vi "Generate Keithley DMM7510 Data.vi"(7 "Previous End":i32, 8 "error in (no error)":errorcluster, 11 "VISA resource name in":refnum<visa-resource-name>) -> (0 "error out":errorcluster, 2 "Graph Data":waveform(dbl)[](array[waveform]), 3 "VISA resource name out":refnum<visa-resource-name>, 4 "Actual sampling time (mean)":dbl, 5 "Current End":i32)   [LabVIEW 2017, in "Acquisition.lvlib"]
doc: "Generates sample waveforms according to the signal type in the HW Config input."
uses:
  Acquisition.lvlib
  <vilib>/Analysis/baseanly.llb/Mean (DBL).vi
  <vilib>/Analysis/NI_AALBase.lvlib
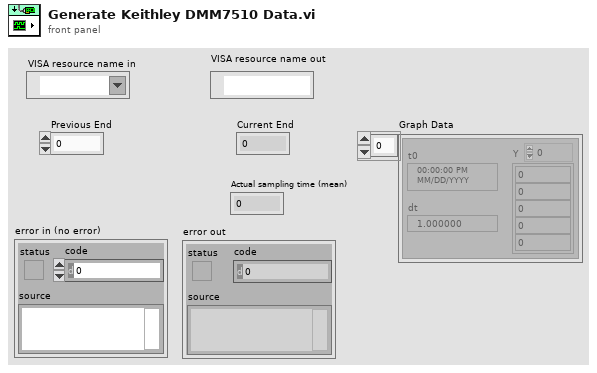
[diagram p1: front panel]
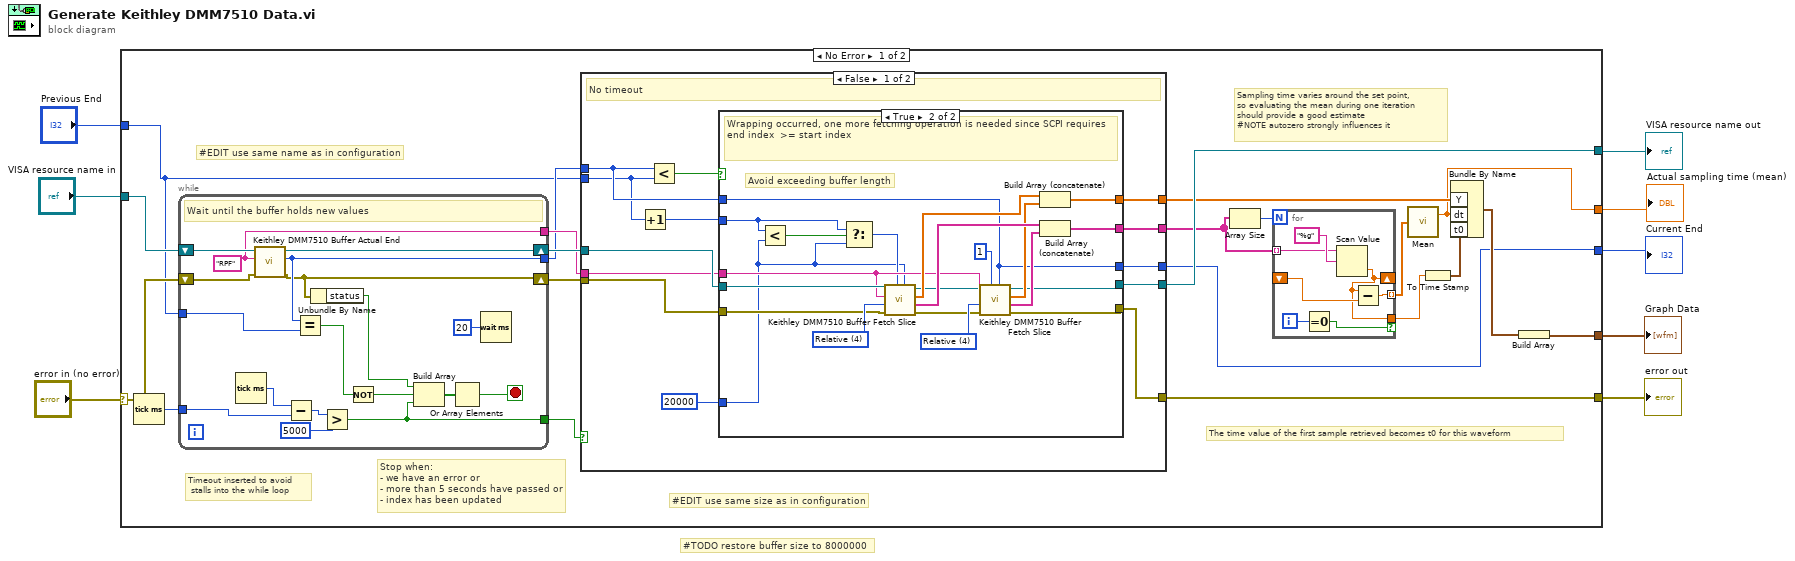
[diagram p0: block diagram]
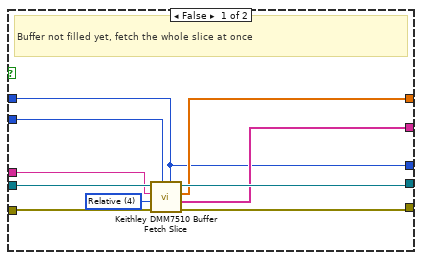
[diagram p2: hidden frame]
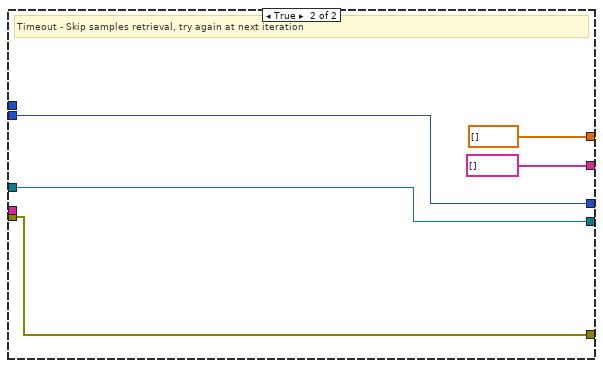
[diagram p3: hidden frame]
diagram:
  # "#TODO restore buffer size to 8000000"
  n1 = case shown="No Error" "error in (no error)" {
    selector: "error in (no error)" -> [w24 w105]
    tunnel: [w22 w105] -> w7
    tunnel: "VISA resource name in" -> [w25 w104]
    tunnel: [w21 w104] -> w5
    tunnel: "Previous End" -> [w23 _]
    tunnel: [w18 _] -> w3
    tunnel: [w17 _] -> w2
    tunnel: [w10 _] -> w1
    frame No Error {
      # "The time value of the first sample retrieved becomes t0 for this waveform"
      # "#EDIT use same name as in configuration"
      # "#EDIT use same size as in configuration"
      # "Timeout inserted to avoid\n stalls into the while loop"
      # "Stop when:\n- we have an error or\n- more than 5 seconds have passed or\n- index has been updated"
      # "Sampling time varies around the set point,\nso evaluating the mean during one iteration\nshould provide a good estimate\n#NOTE autozero strongly influences it"
      n2 = Tick Count (ms)() -> (millisecond timer value=w9:u32)
      n3 = while {
        shift-right: [w46] -> w29
        shift-left: w25 -> [w47]
        shift-right: [w41] -> w28
        shift-left: w24 -> [w45]
        tunnel: [w44] -> w27
        tunnel: [w43] -> w26
        tunnel: w23 -> [w42]
        tunnel: w9 -> [w38]
        tunnel: [w31] -> w14
        stop <- w40 stop-if-true
        w44 = "RPF" ("Buffer Name (defbuffer1)")
        # "Wait until the buffer holds new values"
        n4 = Tick Count (ms)() -> (millisecond timer value=w39:u32)
        n5 = call "Keithley DMM7510 Buffer Actual End.vi"("error in (no error)"=w45, "Buffer Name (defbuffer1)"=w44, "VISA resource name"=w47) -> ("error out"=w41:errorcluster, "Actual End"=w43:i32, "VISA resource name out"=w46:refnum<visa-resource-name>)  [unwired: 6 in]
        n6 = Subtract(x=w39, y=w38) -> (x-y=w37:u32)
        n7 = Equal?(x=w43, y=w42) -> (x = y?=w34:bool)
        n8 = Unbundle By Name(w41) -> ("status"=w32:bool)
        n9 = Greater?(x=w37, y=u32 5000) -> (0:w31:bool)
        n10 = Not(x=w34) -> (.not. x?=w33:bool)
        n11 = Build Array(w32, w33, w31) -> (w35:bool[])
        n12 = Or Array Elements(Boolean array=w35) -> (logical OR=w40:bool)
        n13 = Wait (ms)(milliseconds to wait=u32 20) -> ()  [unwired: 1 out]
      }
      n14 = case shown="False" w14 {
        tunnel: w29 -> [w59 w95]
        tunnel: w28 -> [w58 w96]
        tunnel: w27 -> [w57 _]
        tunnel: w26 -> [w56 _]
        tunnel: w23 -> [w53 w94]
        tunnel: [w52 w96] -> w22
        tunnel: [w51 w95] -> w21
        tunnel: [w50 dbl[] [] ("Measurements")] -> w20
        tunnel: [w49 w94] -> w17
        tunnel: [w48 string[] [] ("Element Value")] -> w15
        frame False {
          # "No timeout"
          n15 = Increment(x=w53) -> (x+1=w55:i32)
          n16 = Less?(x=w56, y=w53) -> (x < y?=w60:bool)
          n17 = case shown="True" w60 {
            tunnel: w58 -> [w69 w80]
            tunnel: w57 -> [w68 w83]
            tunnel: w59 -> [w70 w91]
            tunnel: 20000 ("Buffer Size") -> [_ w72]
            tunnel: [w66 w76] -> w51
            tunnel: [w65 w78] -> w52
            tunnel: [w62 w75] -> w49
            tunnel: w55 -> [w67 w71]
            tunnel: [w64 w90] -> w50
            tunnel: [w63 w89] -> w48
            tunnel: w56 -> [w62 w75]
            frame False {
              w61 = u16 4 items=["Date", "Extra", "Formatted", "Fractional", "Relative", "Seconds", "Status", "Time", "Timestamp", "Unit"] ("Buffer Elements")
              # "Buffer not filled yet, fetch the whole slice at once"
              n18 = call "Keithley DMM7510 Buffer Fetch Slice.vi"("End Index"=w62, "Start Index"=w67, "error in (no error)"=w69, "Buffer Elements"=w61, "Buffer Name"=w68, "VISA resource name"=w70) -> ("error out"=w65:errorcluster, "Element Value"=w63:string[], "Measurements"=w64:dbl[], "VISA resource name out"=w66:refnum<visa-resource-name>)  [unwired: 2 in]
            }
            frame True {
              w81 = u16 4 items=["Date", "Extra", "Formatted", "Fractional", "Relative", "Seconds", "Status", "Time", "Timestamp", "Unit"] ("Buffer Elements")
              w82 = u16 4 items=["Date", "Extra", "Formatted", "Fractional", "Relative", "Seconds", "Status", "Time", "Timestamp", "Unit"] ("Buffer Elements")
              # "Avoid exceeding buffer length"
              # "Wrapping occurred, one more fetching operation is needed since SCPI requires end index  >= start index"
              n19 = Less?(x=w71, y=w72) -> (x < y?=w73:bool)
              n20 = Select(t=w71, s=w73, f=w72) -> (s? t:f=w74:i32)
              n21 = call "Keithley DMM7510 Buffer Fetch Slice.vi"("End Index"=w72, "Start Index"=w74, "error in (no error)"=w80, "Buffer Elements"=w82, "Buffer Name"=w83, "VISA resource name"=w91) -> ("error out"=w79:errorcluster, "Element Value"=w87:string[], "Measurements"=w86:dbl[], "VISA resource name out"=w77:refnum<visa-resource-name>)  [unwired: 2 in]
              n22 = call "Keithley DMM7510 Buffer Fetch Slice.vi"("End Index"=w75, "Start Index"=1, "error in (no error)"=w79, "Buffer Elements"=w81, "Buffer Name"=w83, "VISA resource name"=w77) -> ("error out"=w78:errorcluster, "Element Value"=w88:string[], "Measurements"=w85:dbl[], "VISA resource name out"=w76:refnum<visa-resource-name>)  [unwired: 2 in]
              n23 = Build Array (concatenate)(w86, w85) -> (w90:dbl[])
              n24 = Build Array (concatenate)(w87, w88) -> (w89:string[])
            }
          }
        }
        frame True {
          # "Timeout - Skip samples retrieval, try again at next iteration"
        }
      }
      n25 = Array Size(array=w15) -> (size(s)=w16:i32)
      n26 = for {
        N: w16 -> [_]
        tunnel: w15 -> [w102] mode=indexing
        shift-right: [w99] -> _
        shift-left: _ -> [w101]
        tunnel: [w100] -> w13 mode=indexing
        tunnel: [w99] -> w11 if=w97
        i -> [w98]
        n27 = Equal To 0?(x=w98) -> (x = 0?=w97:bool)
        n28 = Scan Value(string=w102, format string="%g") -> (value=w99:dbl)  [unwired: 1 in, 1 out]
        n29 = Subtract(x=w99, y=w101) -> (x-y=w100:dbl)
      }
      n30 = call-poly <vilib>:"Mean.vi"("X"=w13) -> ("mean"=w10:dbl)  [unwired: 1 out]
      n31 = To Time Stamp(1:w11) -> (0:w12:timestamp)
      n32 = Bundle By Name("Y"=w20, "dt"=w10, "t0"=w12) -> (w19:waveform(dbl))  [unwired: 1 in]
      n33 = Build Array(w19) -> (w18:waveform(dbl)[])
    }
    frame Error {
    }
  }
  "error out" <- w7
  "Graph Data" <- w3
  "VISA resource name out" <- w5
  "Current End" <- w2
  "Actual sampling time (mean)" <- w1
